vi "Save Project.vi"(8 "error in (no error)":errorcluster, 10 "Path (empty)":path, 11 "Project in":refnum<vi>) -> (0 "error out":errorcluster, 3 "Project out":refnum<vi>)   [LabVIEW 2019, in "VI Scripting Tools.lvlib"]
uses:
  VI Scripting Tools.lvlib
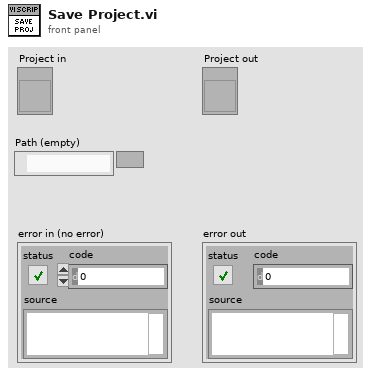
[diagram p1: front panel]
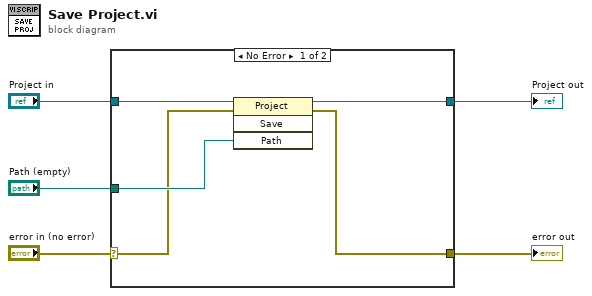
[diagram p0: block diagram]
diagram:
  n1 = case shown="No Error" "error in (no error)" {
    selector: "error in (no error)" -> [w6 w11]
    tunnel: [w10 w11] -> w5
    tunnel: [w9 w12] -> w4
    tunnel: "Project in" -> [w8 w12]
    tunnel: "Path (empty)" -> [w7 _]
    frame No Error {
      n2 = invoke class="Project" method="Save"(reference=w8, error in=w6, "Path"=w7) -> (reference out=w9:refnum<vi>, error out=w10:errorcluster)  [unwired: 1 in, 2 out]
    }
    frame Error {
    }
  }
  "error out" <- w5
  "Project out" <- w4
